vi "Completion Notification Msg.vi"() -> ()   [LabVIEW 2023, in "Async Methods Actor.lvlib"]
uses:
  Async Methods Actor.lvlib
  Async Methods Actor Messages/Completion Notification Msg/Completion Notification Msg.lvclass
panel:
  in  "Completion Notification Msg.lvclass":refnum<class "Completion Notification Msg.lvclass">
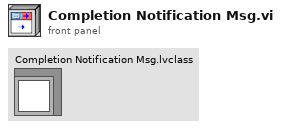
[diagram p1: front panel]
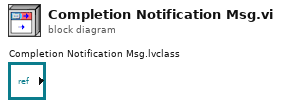
[diagram p0: block diagram]
diagram:
